vi "SQL_Table_Test_Count.vi"() -> (3 "Data":string[][](array[string]))   [LabVIEW 2014]
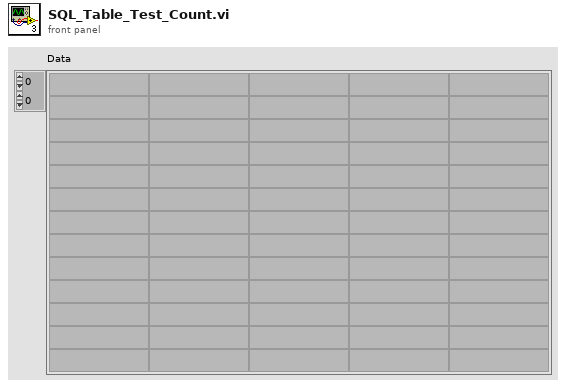
[diagram p1: front panel]
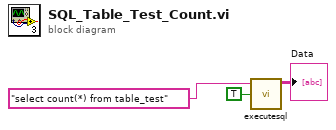
[diagram p0: block diagram]
diagram:
  n1 = call "executesql.vi"("Return Data (T)"=TRUE, "Command Text"="select count(*) from table_test") -> ("Data"=→"Data":string[][])  [unwired: 5 in, 1 out]
